vi "Load.vi"(4 "Index":i32, 7 "SDC":string, 8 "error in (no error)":errorcluster, 9 "VISA":refnum<visa-resource-name>, 10 "DeviceName":string, 11 "DBRefNum":i32) -> (0 "error out":errorcluster)   [LabVIEW 2020, in "ModBus Serial Master.lvlib"]
doc: "加载ModBus TCP Master进程"
uses:
  ModBus Serial Master.lvlib
  CCTM/CCT.ctl
  CCTM.lvlib
  ModBusCommon.lvlib
panel:
  in  "Debug":bool
  in  "POLL":bool
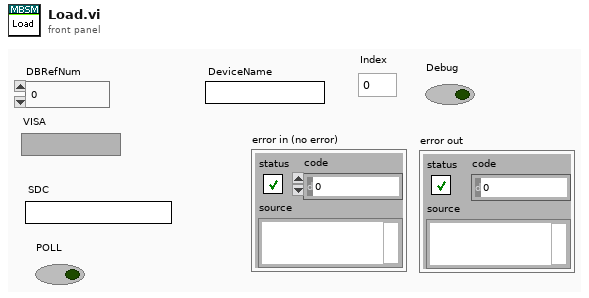
[diagram p1: front panel]
types:
  T1 = typedef "CCTM.lvlib/CCT.ctl" = cluster{"Connected Name":string, "Connection Reference":refnum<vi>, "Device Index":i32, "DriverName":string, "Register Number":i32}
  T2 = enum32{"Invalid", "Standard", "Closed", "Hidden", "Minimized", "Maximized"}
  T3 = typedef "DriverCommon.lvlib/Swap.ctl" = enum16{"No Change", "Swap"}
  T4 = typedef "DriverCommon.lvlib/MB Modbus Command.ctl" = cluster{"Function Code":u8, "Starting Address":u16, "Quantity":u16, "Data":u16[], "Discrete":bool[], "Index of Tags":i32[]}
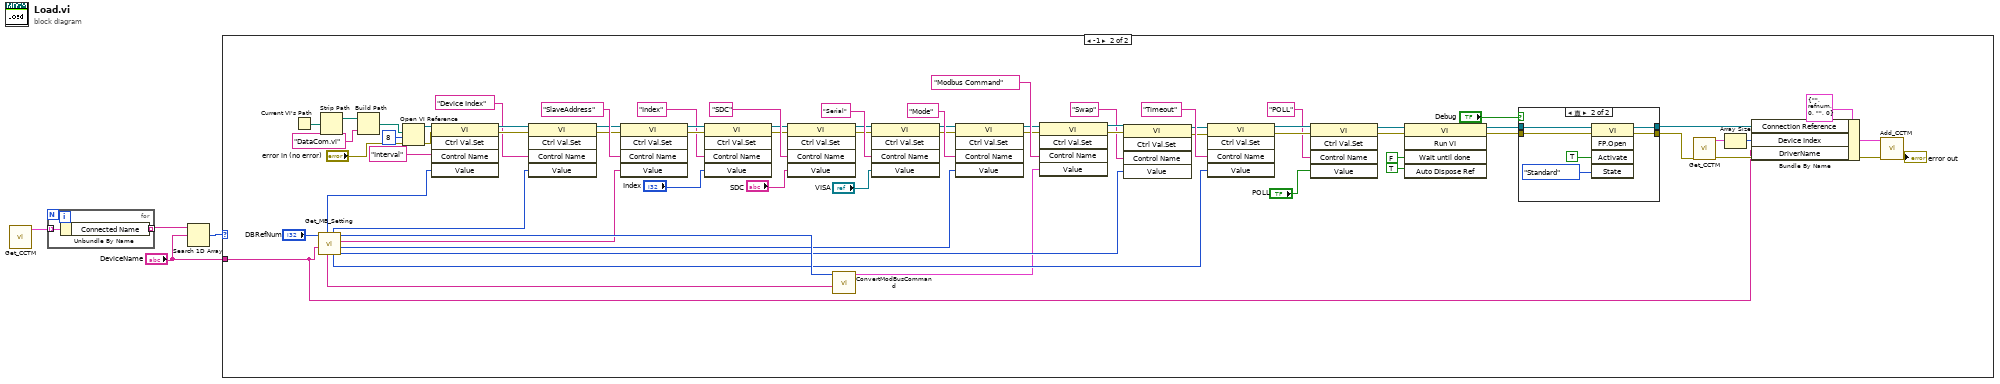
[diagram p0: block diagram]
diagram:
  n1 = call "Get_CCTM.vi"() -> ("All Connections"=w3:T1[])  [unwired: 10 in, 1 out]
  n2 = for {
    tunnel: w3 -> [w6] mode=indexing
    tunnel: [w5] -> w4 mode=indexing
    n3 = Unbundle By Name(w6) -> ("Connected Name"=w5:string)
  }
  n4 = Search 1D Array(1D array=w4, element="DeviceName") -> (index of element=w1:i32)  [unwired: 1 in]
  n5 = case shown="-1" w1 {
    tunnel: "DeviceName" -> [_ w13]
    frame 0, Default {
    }
    frame -1 {
      n6 = Current VI's Path() -> (path=w61:path)
      n7 = call "Get_MB_Setting.vi"("DeviceName"=w13, "DBRefNum"="DBRefNum") -> ("Swap"=w67:T3, "Mode"=w69:enum16{"RTU", "ASCII"}, "Address"=w73:string, "DBRefNum Out"=w74:i32, "Timeout"=w70:i32, "Device Index"=w7:u8, "Name"=w72:string, "Interval"=w68:u32)  [unwired: 2 in]
      n8 = Strip Path(path=w61) -> (stripped path=w60:path)  [unwired: 1 out]
      n9 = Build Path(base path=w60, name or relative path="DataCom.vi") -> (appended path=w58:path)
      n10 = Open VI Reference(vi path=w58, options=8, error in (no error)="error in (no error)") -> (vi reference=w45:refnum<vi>, error out=w44:errorcluster)  [unwired: 3 in]
      n11 = invoke class="VI" method="Ctrl Val.Set"(reference=w45, error in=w44, "Control Name"="Interval", "Value"=w68) -> (reference out=w12:refnum<vi>, error out=w10:errorcluster)  [unwired: 1 in, 3 out]
      n12 = invoke class="VI" method="Ctrl Val.Set"(reference=w12, error in=w10, "Control Name"="Device Index", "Value"=w7) -> (reference out=w11:refnum<vi>, error out=w9:errorcluster)  [unwired: 1 in, 3 out]
      n13 = invoke class="VI" method="Ctrl Val.Set"(reference=w11, error in=w9, "Control Name"="SlaveAddress", "Value"=w73) -> (reference out=w42:refnum<vi>, error out=w40:errorcluster)  [unwired: 1 in, 3 out]
      n14 = invoke class="VI" method="Ctrl Val.Set"(reference=w42, error in=w40, "Control Name"="Index", "Value"="Index") -> (reference out=w41:refnum<vi>, error out=w39:errorcluster)  [unwired: 1 in, 3 out]
      n15 = invoke class="VI" method="Ctrl Val.Set"(reference=w41, error in=w39, "Control Name"="SDC", "Value"="SDC") -> (reference out=w49:refnum<vi>, error out=w48:errorcluster)  [unwired: 1 in, 3 out]
      n16 = call "ConvertModBusCommand.vi"("DeviceName"=w72, "DB Reference In"=w74) -> ("Modbus Command"=w25:T4[])  [unwired: 9 in]
      n17 = invoke class="VI" method="Ctrl Val.Set"(reference=w49, error in=w48, "Control Name"="Serial", "Value"="VISA") -> (reference out=w54:refnum<vi>, error out=w53:errorcluster)  [unwired: 1 in, 3 out]
      n18 = invoke class="VI" method="Ctrl Val.Set"(reference=w54, error in=w53, "Control Name"="Mode", "Value"=w69) -> (reference out=w57:refnum<vi>, error out=w56:errorcluster)  [unwired: 1 in, 3 out]
      n19 = invoke class="VI" method="Ctrl Val.Set"(reference=w57, error in=w56, "Control Name"="Modbus Command", "Value"=w25) -> (reference out=w36:refnum<vi>, error out=w34:errorcluster)  [unwired: 1 in, 3 out]
      n20 = invoke class="VI" method="Ctrl Val.Set"(reference=w36, error in=w34, "Control Name"="Swap", "Value"=w67) -> (reference out=w35:refnum<vi>, error out=w33:errorcluster)  [unwired: 1 in, 3 out]
      n21 = invoke class="VI" method="Ctrl Val.Set"(reference=w35, error in=w33, "Control Name"="Timeout", "Value"=w70) -> (reference out=w31:refnum<vi>, error out=w30:errorcluster)  [unwired: 1 in, 3 out]
      n22 = invoke class="VI" method="Ctrl Val.Set"(reference=w31, error in=w30, "Control Name"="POLL", "Value"="POLL") -> (reference out=w29:refnum<vi>, error out=w28:errorcluster)  [unwired: 1 in, 3 out]
      n23 = invoke class="VI" method="Run VI"(reference=w29, error in=w28, "Wait until done"=FALSE ("Wait Until Done"), "Auto Dispose Ref"=TRUE ("Auto Dispose Reference")) -> (reference out=w20:refnum<vi>, error out=w19:errorcluster)  [unwired: 1 in, 3 out]
      n24 = case shown="真" "Debug" {
        tunnel: w20 -> [w77 w83]
        tunnel: w19 -> [w76 w82]
        tunnel: [w76 w79] -> w17
        tunnel: [w77 w78] -> w16
        frame False {
        }
        frame True {
          n25 = invoke class="VI" method="FP.Open"(reference=w83, error in=w82, "Activate"=TRUE ("Activate?"), "State"=T2."Standard") -> (reference out=w78:refnum<vi>, error out=w79:errorcluster)  [unwired: 1 in, 3 out]
        }
      }
      n26 = call "Get_CCTM.vi"("error in (no error)"=w17) -> ("error out"=w21:errorcluster, "All Connections"=w23:T1[])  [unwired: 9 in]
      n27 = Array Size(array=w23) -> (size(s)=w22:i32)
      n28 = Bundle By Name(cluster=T1 {"Connected Name"="", "Connection Reference"=refnum, "Device Index"=0, "DriverName"="", "Register Number"=0} ("New/Delete Connection"), "Connection Reference"=w16, "Device Index"=w22, "DriverName"=w13) -> (w24:T1)
      n29 = call "Add_CCTM.vi"("error in (no error)"=w21, "New/Delete Connection"=w24) -> ("error out"=→"error out":errorcluster)  [unwired: 9 in]
    }
  }
